vi "REACTOR_PARSE_REPETICIONES.vi"(11 "String":string="Numero de repeticiones: 5") -> (1 "#REPETICIONES":i32=1)   [LabVIEW 2017]
panel:
  # "Numero de repeticiones: 5"
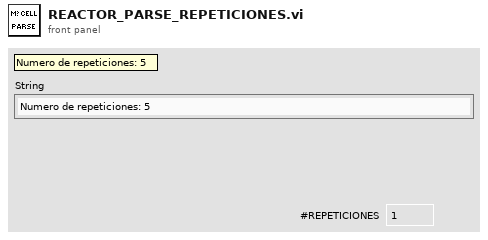
[diagram p1: front panel]
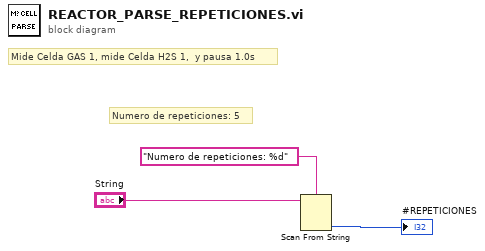
[diagram p0: block diagram]
diagram:
  # "Mide Celda GAS 1, mide Celda H2S 1,  y pausa 1.0s"
  # "Numero de repeticiones: 5"
  n1 = Scan From String(format string="Numero de repeticiones: %d", input string="String") -> (output 1=→"#REPETICIONES":i32)  [unwired: 3 in, 3 out]
